vi "Channel_name_checker.vi"(2 "Email On Error?":bool, 3 "Channel names":string[](array[string])) -> (0 "No of Errors":i32, 1 "Channel names Out":string[](array[string]))   [LabVIEW 2020]
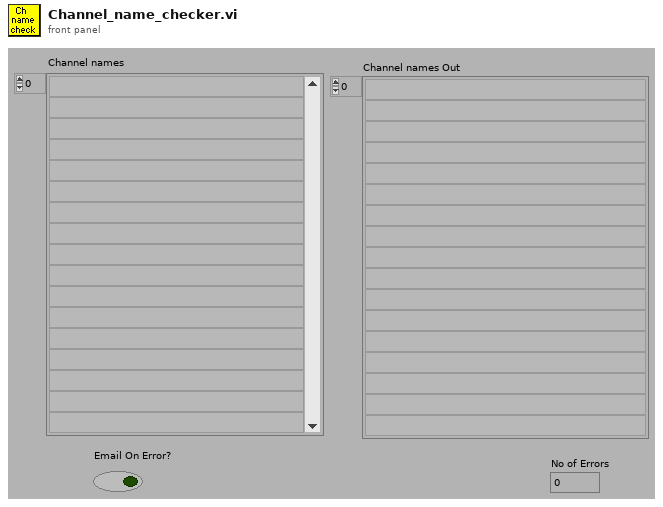
[diagram p1: front panel]
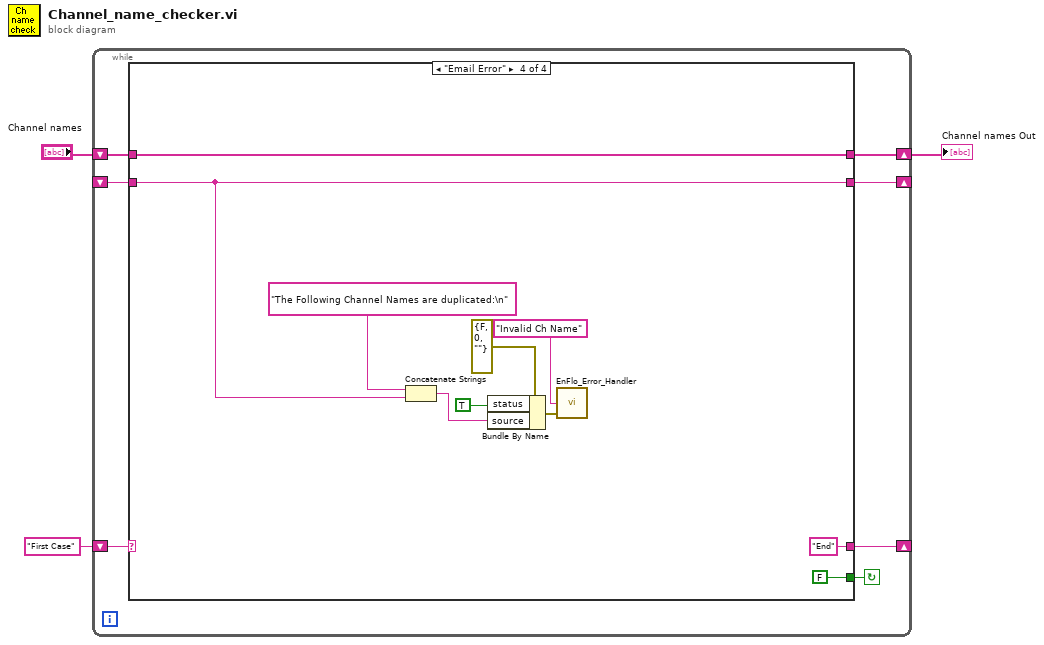
[diagram p0: block diagram]
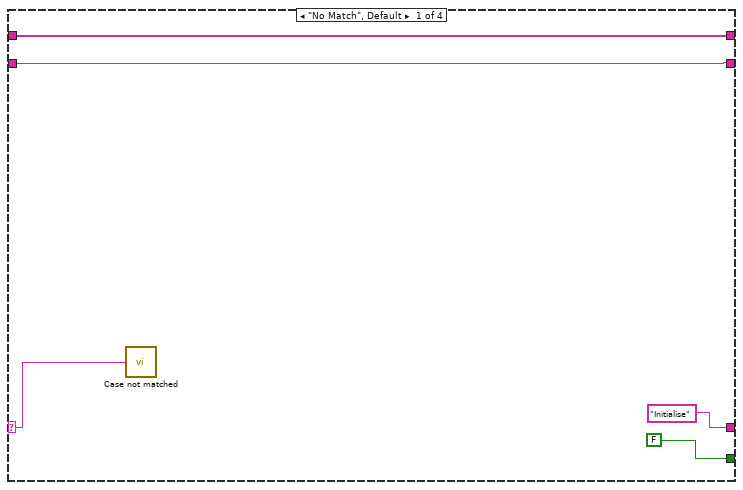
[diagram p2: hidden frame]
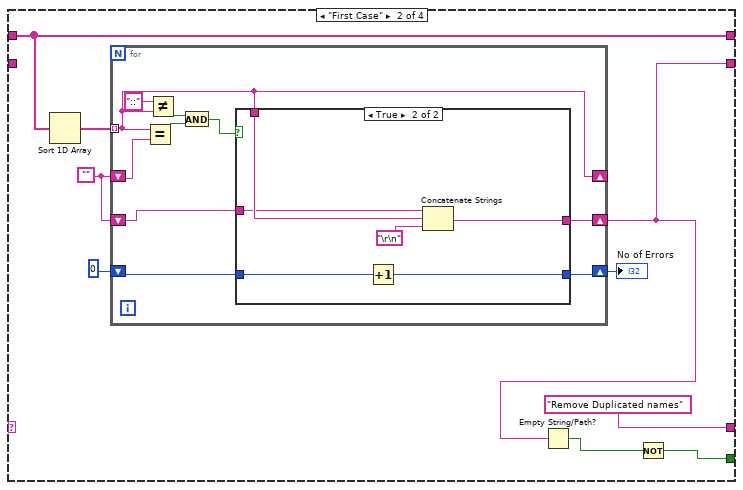
[diagram p3: hidden frame]
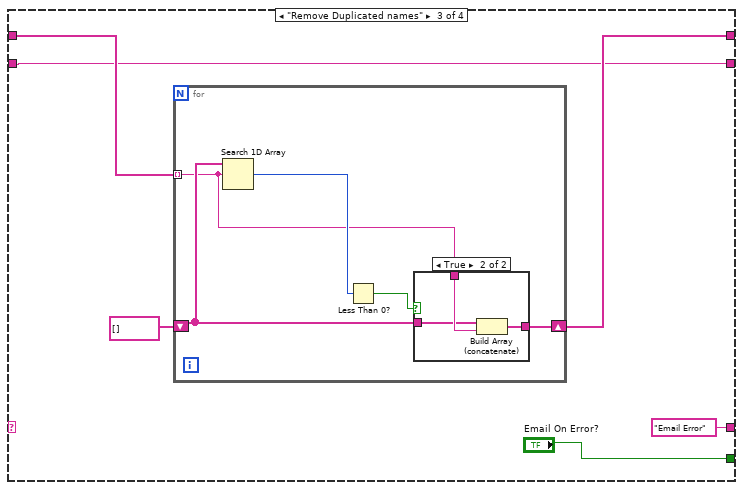
[diagram p5: hidden frame]
diagram:
  n1 = while {
    shift-left: "First Case" -> [w8]
    shift-right: [w9] -> _
    shift-right: [w5] -> w1
    shift-left: "Channel names" -> [w7]
    shift-right: [w6] -> _
    shift-left: _ -> [w4]
    stop <- w10 continue-if-true
    n2 = case shown="\"Email Error\"" w8 {
      selector: w8 -> [w11 _ _ _]
      tunnel: [FALSE w16 "Email On Error?" FALSE ("Email On Error?")] -> w10
      tunnel: ["Initialise" "Remove Duplicated names" "Email Error" "End"] -> w9
      tunnel: w7 -> [w13 w19 w47 w60]
      tunnel: [w12 w18 w45 w61] -> w6
      tunnel: [w13 w19 w46 w60] -> w5
      tunnel: w4 -> [w12 _ w45 w61]
      frame "No Match", Default {
        n3 = call "Case not matched.vi"("Case Name not Matched"=w11) -> ()
      }
      frame "First Case" {
        w23 = ""
        n4 = Sort 1D Array(array=w19) -> (sorted array=w20:string[])
        n5 = for {
          shift-right: [w33] -> _
          shift-left: w23 -> [w34]
          tunnel: w20 -> [w33] mode=indexing
          shift-right: [w27] -> w22
          shift-left: 0 -> [w28]
          shift-right: [w25] -> w18
          shift-left: w23 -> [w26]
          n6 = Equal?(x=w33, y=w34) -> (x = y?=w30:bool)
          n7 = Not Equal?(x="::", y=w33) -> (x != y?=w31:bool)
          n8 = And(x=w31, y=w30) -> (x .and. y?=w29:bool)
          n9 = case shown="True" w29 {
            tunnel: w33 -> [_ w40]
            tunnel: w28 -> [w36 w42]
            tunnel: [w36 w41] -> w27
            tunnel: w26 -> [w35 w39]
            tunnel: [w35 w38] -> w25
            frame False {
            }
            frame True {
              n10 = Increment(x=w42) -> (x+1=w41:i32)
              n11 = Concatenate Strings(w39, w40, "\r\n") -> (w38:string)
            }
          }
        }
        "No of Errors" <- w22
        n12 = Empty String/Path?(string/path=w18) -> (empty?=w17:bool)
        n13 = Not(x=w17) -> (.not. x?=w16:bool)
      }
      frame "Remove Duplicated names" {
        n14 = for {
          shift-right: [w53] -> w46
          shift-left: string[] [] -> [w52]
          tunnel: w47 -> [w49] mode=indexing
          n15 = Search 1D Array(1D array=w52, element=w49) -> (index of element=w51:i32)  [unwired: 1 out]
          n16 = Less Than 0?(x=w51) -> (x < 0?=w50:bool)
          n17 = case shown="True" w50 {
            tunnel: w49 -> [_ w57]
            tunnel: [w54 w56] -> w53
            tunnel: w52 -> [w54 w55]
            frame False {
            }
            frame True {
              n18 = Build Array (concatenate)(w55, w57) -> (w56:string[])
            }
          }
        }
      }
      frame "Email Error" {
        n19 = Concatenate Strings("The Following Channel Names are duplicated:\n", w61) -> (w65:string)
        n20 = Bundle By Name(cluster=errorcluster {"status"=FALSE, "code"=0, "source"=""} ("error in (no error)"), "status"=TRUE ("Bundle Element"), "source"=w65) -> (w64:errorcluster)
        n21 = call "EnFlo_Error_Handler.vi"("error in (no error)"=w64, "Error Type"="Invalid Ch Name") -> ()  [unwired: 1 in, 3 out]
      }
    }
  }
  "Channel names Out" <- w1
